vi "N6705B_Dlog_record.vi"(4 "Number of cycles":i32, 5 "Log?":bool, 7 "Data Log Period (0.1 s)":dbl=1.0 format="%#_13g", 8 "error in (no error)":errorcluster {"code" format="%.0x"}, 9 "N":string, 10 "Data Log File Path (data1.dlog)":string="Charge.dlog", 11 "VISA resource name":refnum<visa-resource-name>="VAL_N6705B") -> (0 "error out":errorcluster {"code" format="%.0x"}, 2 "File Name Out":string, 3 "VISA resource name out":refnum<visa-resource-name>)   [LabVIEW 2015]
uses:
  <instrlib>/Agilent N6700 Series/Agilent N6700 Series.lvlib
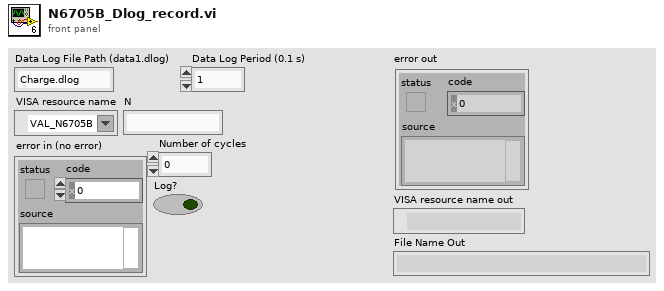
[diagram p1: front panel]
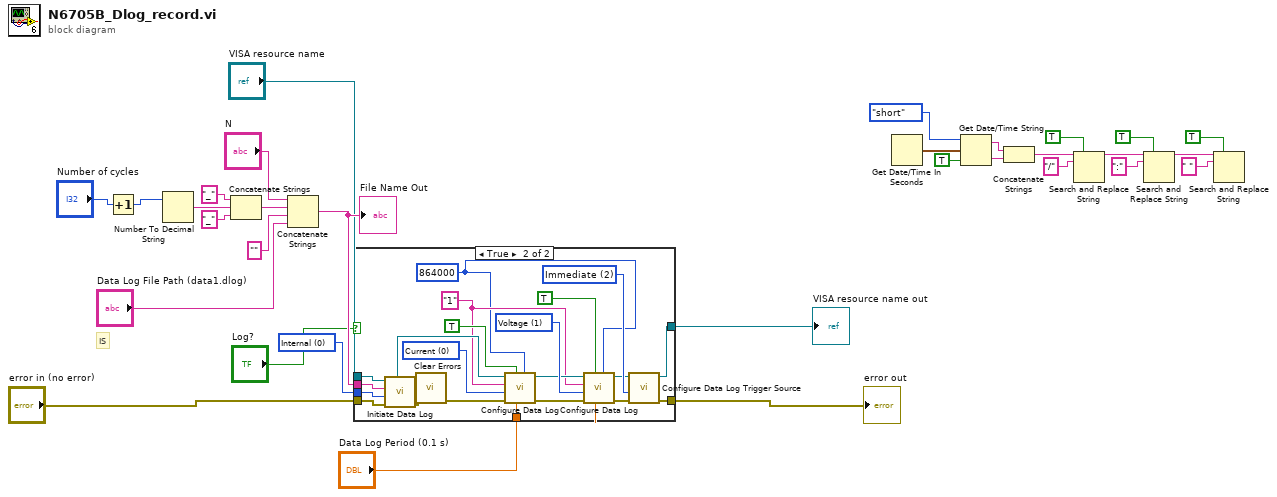
[diagram p0: block diagram]
diagram:
  w18 = 0 items=["Internal", "External"] ("Location (0: Internal)")
  # "IS"
  n1 = Increment(x="Number of cycles") -> (x+1=w2:i32)
  n2 = Number To Decimal String(number=w2) -> (decimal integer string=w6:string)  [unwired: 1 in]
  n3 = Concatenate Strings("_" ("string"), w6, "_" ("string")) -> (w8:string)
  n4 = Concatenate Strings("N", w8, "" ("string"), "Data Log File Path (data1.dlog)") -> (w17:string)
  "File Name Out" <- w17
  n5 = case shown="True" "Log?" {
    tunnel: w18 -> [_ w48]
    tunnel: w17 -> [_ w47]
    tunnel: "VISA resource name" -> [w33 w46]
    tunnel: "error in (no error)" -> [w32 w45]
    tunnel: [w32 w44] -> w14
    tunnel: [w33 w43] -> w13
    tunnel: "Data Log Period (0.1 s)" -> [_ w37]
    frame False {
    }
    frame True {
      w42 = 1 items=["Voltage"=1, "Current"=0] ("Data Log Type (1: Voltage)")
      w49 = 2 items=["External", "Software", "Immediate", "Voltage1", "Voltage2", "Voltage3", "Voltage4", "Current1", "Current2", "Current3", "Current4"] ("Data Log Trigger Source (2: Immediate)")
      w34 = 864000 ("Data Log Duration (30 s)")
      w50 = 0 items=["Voltage"=1, "Current"=0] ("Data Log Type (1: Voltage)")
      w38 = "1" ("Channel Name (1)")
      n6 = call <instrlib>:"Initiate Data Log.vi"("error in (no error)"=w45, "Location (0: Internal)"=w48, "Data Log File Path (data1.dlog)"=w47, "VISA resource name"=w46) -> ("error out"=w53:errorcluster, "VISA resource name out"=w52:refnum<visa-resource-name>)  [unwired: 6 in]
      n7 = call <vilib>:"Clear Errors.vi"("error in (no error)"=w53) -> ("error out"=w54:errorcluster)  [unwired: 5 in, 1 out]
      n8 = call <instrlib>:"Configure Data Log.vi"("Data Log Duration (30 s)"=w34, "Data Log Period (0.1 s)"=w37, "Enable Data Log (True)"=TRUE, "error in (no error)"=w54, "Data Log Type (1: Voltage)"=w50, "Channel Name (1)"=w38, "VISA resource name"=w52) -> ("error out"=w40:errorcluster, "VISA resource name out"=w41:refnum<visa-resource-name>)  [unwired: 3 in]
      n9 = call <instrlib>:"Configure Data Log.vi"("Data Log Duration (30 s)"=w34, "Data Log Period (0.1 s)"=w37, "Enable Data Log (True)"=TRUE, "error in (no error)"=w40, "Data Log Type (1: Voltage)"=w42, "Channel Name (1)"=w38, "VISA resource name"=w41) -> ("error out"=w35:errorcluster, "VISA resource name out"=w36:refnum<visa-resource-name>)  [unwired: 3 in]
      n10 = call <instrlib>:"Configure Data Log Trigger Source.vi"("error in (no error)"=w35, "Data Log Trigger Source (2: Immediate)"=w49, "VISA resource name"=w36) -> ("error out"=w44:errorcluster, "VISA resource name out"=w43:refnum<visa-resource-name>)  [unwired: 7 in]
    }
  }
  "error out" <- w14
  "VISA resource name out" <- w13
  n11 = Get Date/Time In Seconds() -> (seconds since 1Jan1904=w19:timestamp)
  n12 = Get Date/Time String(date format (0)=enum16{"short", "long", "abbreviated"}."short", seconds (now)=w19, want seconds? (F)=TRUE) -> (date string=w20:string, time string=w21:string)
  n13 = Concatenate Strings(w20, w21) -> (w23:string)
  n14 = Search and Replace String(replace all?=TRUE ("replace all? (F)"), input string=w23, search string="/") -> (result string=w28:string)  [unwired: 5 in, 3 out]
  n15 = Search and Replace String(replace all?=TRUE ("replace all? (F)"), input string=w28, search string=":") -> (result string=w31:string)  [unwired: 5 in, 3 out]
  n16 = Search and Replace String(replace all?=TRUE ("replace all? (F)"), input string=w31, search string=" ") -> ()  [unwired: 5 in, 4 out]
